vi "resume-from-progress.vi"(8 "current slice reference":refnum<vi>, 9 "name or relative path":string, 10 "desired number of pages":i32, 11 "Data TIFF File":path) -> (1 "number of pages recovered":i32, 3 "new tiff pointer":i64 format="%x")   [LabVIEW 2013]
uses:
  imagereconstruction/x64/Debug/labviewdll.dll
panel:
  out "whole match":string
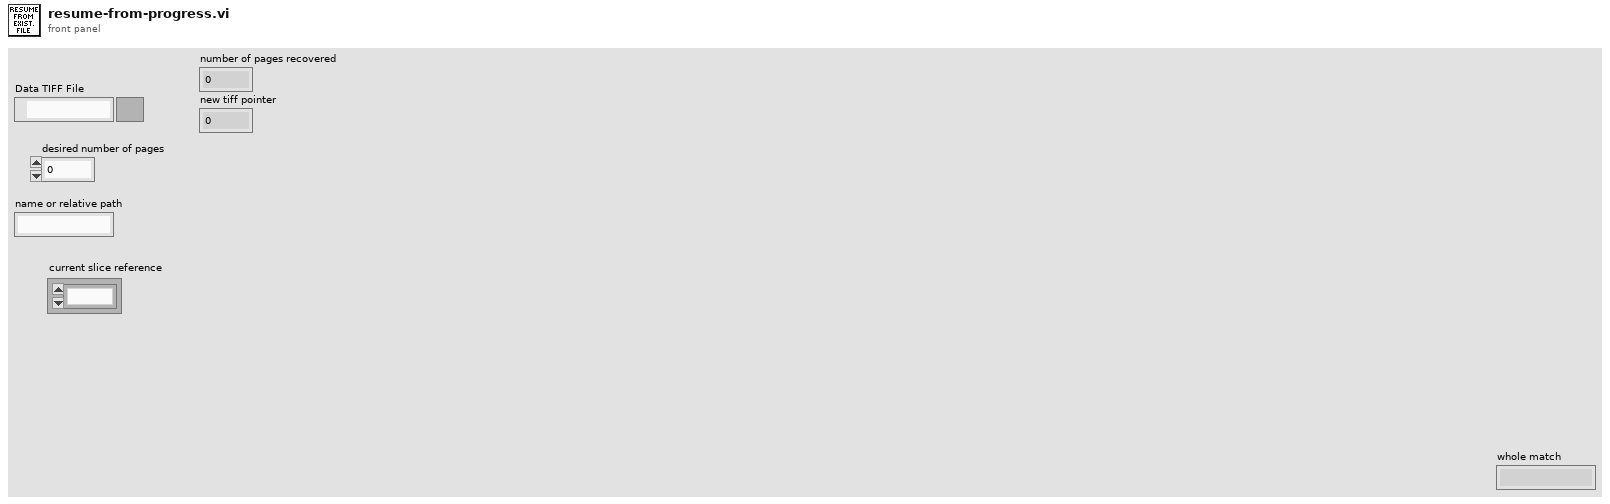
[diagram p1: front panel]
types:
  T1 = typedef "tags_cluster.ctl" = cluster{"compression":i32, "image width":i32, "image length":i32, "host computer":string, "software":string, "bitness":i32, "number of pages":i32, "samples per pixel":i32, "scanline size":i32, "strip size":i32, "lines per strip":i32}
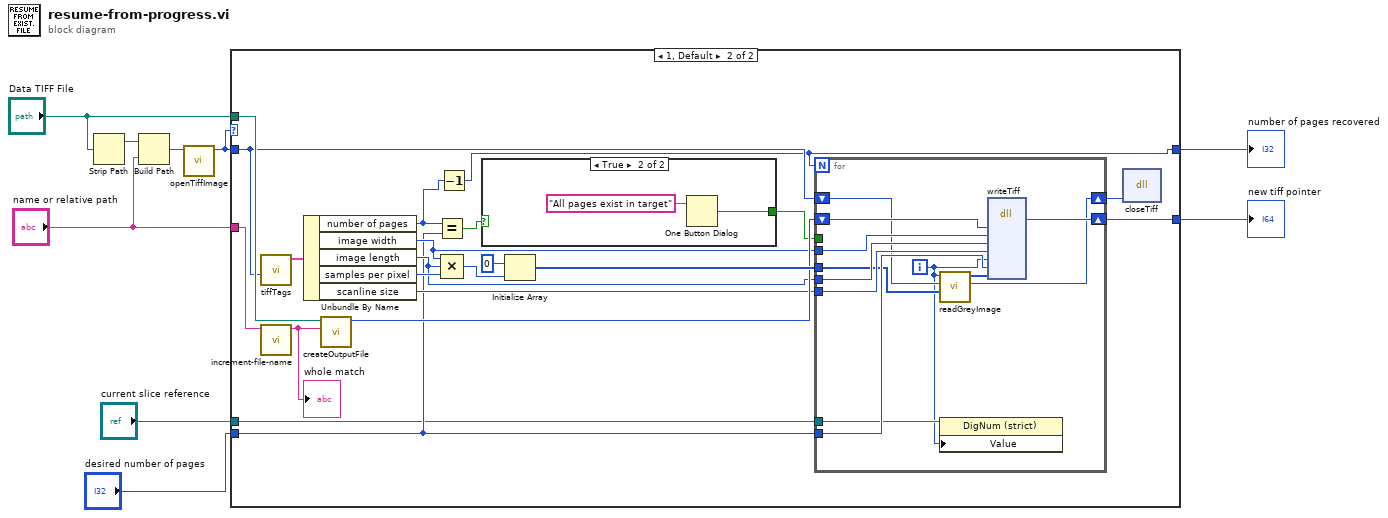
[diagram p0: block diagram]
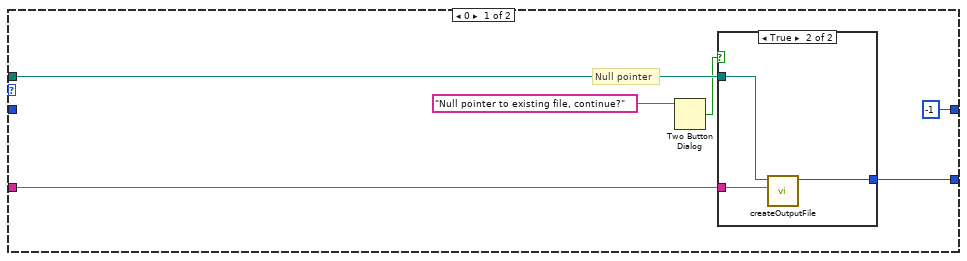
[diagram p2: hidden frame]
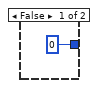
[diagram p3: hidden frame]
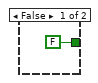
[diagram p4: hidden frame]
diagram:
  n1 = Strip Path(path="Data TIFF File") -> (stripped path=w9:path)  [unwired: 1 out]
  n2 = Build Path(base path=w9, name or relative path="name or relative path") -> (appended path=w8:path)
  n3 = call "openTiffImage.vi"("Path string"=w8) -> ("returned pointer"=w7:i64)  [unwired: 9 in, 1 out]
  n4 = case shown="1, Default" w7 {
    tunnel: w7 -> [_ w33]
    tunnel: "name or relative path" -> [w14 w39]
    tunnel: "Data TIFF File" -> [w15 w37]
    tunnel: [w13 w27] -> w1
    tunnel: [-1 ("number of pages") w20] -> w4
    tunnel: "desired number of pages" -> [_ w25]
    tunnel: "current slice reference" -> [_ w22]
    frame 0 {
      # "Null pointer"
      n5 = Two Button Dialog(message="Null pointer to existing file, continue?") -> (T button?=w11:bool)  [unwired: 2 in]
      n6 = case shown="True" w11 {
        tunnel: w15 -> [_ w19]
        tunnel: w14 -> [_ w18]
        tunnel: [0 w17] -> w13
        frame False {
        }
        frame True {
          n7 = call "createOutputFile.vi"("name or relative path"=w18, "Data TIFF File"=w19) -> ("new tiff pointer"=w17:i64)  [unwired: 9 in]
        }
      }
    }
    frame 1, Default {
      n8 = call "tiffTags.vi"("tif pointer"=w33) -> ("Image Properties"=w40:T1)  [unwired: 8 in, 2 out]
      n9 = call "increment-file-name.vi"("name or relative path"=w39) -> ("concatenated string"=w38:string)  [unwired: 10 in]
      "whole match" <- w38
      n10 = Unbundle By Name(w40) -> ("number of pages"=w21:i32, "image width"=w30:i32, "image length"=w29:i32, "samples per pixel"=w36:i32, "scanline size"=w28:i32)
      n11 = call "createOutputFile.vi"("name or relative path"=w38, "Data TIFF File"=w37) -> ("new tiff pointer"=w31:i64)  [unwired: 9 in]
      n12 = Equal?(x=w21, y=w25) -> (x = y?=w24:bool)
      n13 = Decrement(x=w21) -> (x-1=w20:i32)
      n14 = Compound Arithmetic op=MULTIPLY(w30, w29, w36) -> (w35:i32)
      n15 = case shown="True" w24 {
        tunnel: [FALSE ("true") w42] -> w23
        frame False {
        }
        frame True {
          n16 = One Button Dialog(message="All pages exist in target") -> (true=w42:bool)  [unwired: 1 in]
        }
      }
      n17 = Initialize Array(u8 0 ("element"), w35) -> (w32:u8[])
      n18 = for {
        N: w20 -> [_]
        tunnel: w32 -> [w48]
        shift-right: [w44] -> w26
        shift-left: w33 -> [w47]
        tunnel: w30 -> [w54]
        tunnel: w29 -> [w53]
        tunnel: w28 -> [w52]
        tunnel: w25 -> [w51]
        shift-right: [w50] -> w27
        shift-left: w31 -> [w55]
        tunnel: w23 -> [_]
        tunnel: w22 -> [w49]
        i -> [w46]
        n19 = call "readGreyImage.vi"("raster"=w48, "tif"=w47, "Image Number"=w46) -> ("tif pointer"=w44:i64, "pixels"=w45:u8[])  [unwired: 5 in, 2 out]
        n20 = property class="DigNum (strict)"(reference=w49, "Value"=w46) -> ()  [unwired: 1 in, 2 out]
        n21 = dll-call lib="D:/work/uni/FYP/reconrepo/imagereconstruction/x64/Debug/labviewdll.dll" fn="writeTiff"("resultTif"=w55, "w"=w54, "l"=w53, "scanlineSize"=w52, "page"=w46, "npages"=w51, "data"=w45) -> ("return type"=w50:i64)  [unwired: 10 in, 2 out]
      }
      n22 = dll-call lib="D:/work/uni/FYP/reconrepo/imagereconstruction/x64/Debug/labviewdll.dll" fn="closeTiff"("tiff"=w26) -> ()  [unwired: 5 in, 2 out]
    }
  }
  "new tiff pointer" <- w1
  "number of pages recovered" <- w4
